vi "Image_Save_Handler_v_01.vi"(6 "Stop":bool, 8 "Sample+1":bool, 9 "Sample Name":string="Test Sample", 10 "Cam2":T2, 11 "Cam1":T2) -> (0 "Last Image?":bool, 2 "Image2":T1, 3 "Image1":T1)   [LabVIEW 2019]
doc: "Saves every 6th image in a sub folder in the current directory (specified from Sample Name). When a true is sent to Sample+1 a new subfolder is created with incremental numbering.\nExample of folders: \n../images/Sample_Name/Sample_Name1\n../images/Sample_Name/Sample_Name2"
uses:
  <extravilib>/ChannelInstances/Stream-t'IMAQ Image.ctl'/)Channel.ctl
  <vilib>/vision/Image Controls.llb/IMAQ Image.ctl
  <extravilib>/ChannelInstances/Stream-t'IMAQ Image.ctl'/Read With Abort.vi
  <extravilib>/ChannelInstances/Stream-t'IMAQ Image.ctl'/EndpointRead.vi
  <extravilib>/ChannelInstances/Stream-t'IMAQ Image.ctl'/)Channel.vi
  <resource>/ChannelSupport/_ChannelSupport/WaitIfNeeded.vi
  <extravilib>/ChannelInstances/Stream-t'IMAQ Image.ctl'.lvlib
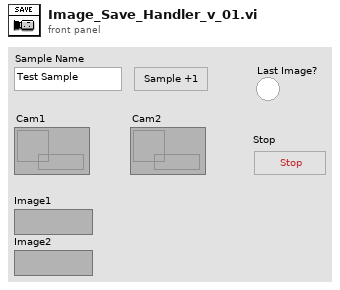
[diagram p1: front panel]
types:
  T1 = typedef "IMAQ Image.ctl" = refnum<image>
  T2 = typedef "Stream-t'IMAQ Image.ctl'.lvlib/)Channel.ctl" = refnum<queue>
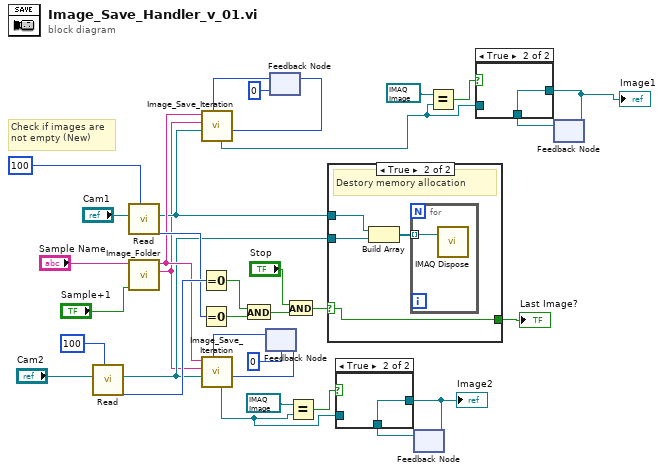
[diagram p0: block diagram]
diagram:
  # "Check if images are\nnot empty (New)"
  n1 = call <extravilib>:"Read.vi"("timeout in ms (-1)"=100, "channel"="Cam2") -> ("element"=w18:T1, "count"=w29:i32)  [unwired: 5 in, 3 out]
  n2 = call <extravilib>:"Read.vi"("timeout in ms (-1)"=100, "channel"="Cam1") -> ("element"=w19:T1, "count"=w21:i32)  [unwired: 5 in, 3 out]
  n3 = call "Image_Folder.vi"("New sample"="Sample+1", "Sample Name"="Sample Name") -> ("Subfolder Name"=w1:string, "Subfolder Path"=w20:string)  [unwired: 8 in]
  n4 = Equal To 0?(x=w29) -> (x = 0?=w24:bool)
  n5 = Equal To 0?(x=w21) -> (x = 0?=w23:bool)
  n6 = And(x=w24, y=w23) -> (x .and. y?=w22:bool)
  n7 = feedback #1(0 ("Iteration count out")) -> (w13:i32)
  n8 = call "Image_Save_Iteration.vi"("Iteration count in"=w13, "Image"=w18, "Subfolder Name"=w1, "Subfolder path"=w20) -> ("Iteration count out"=w14:i32, "Imageout"=w9:T1)  [unwired: 5 in, 1 out]
  n9 = feedback-in #1(w14) -> ()
  n10 = feedback #2(0 ("Iteration count out")) -> (w16:i32)
  n11 = call "Image_Save_Iteration.vi"("Iteration count in"=w16, "Image"=w19, "Subfolder Name"=w1, "Subfolder path"=w20) -> ("Iteration count out"=w17:i32, "Imageout"=w2:T1)  [unwired: 5 in, 1 out]
  n12 = feedback-in #2(w17) -> ()
  n13 = And(x="Stop", y=w22) -> (x .and. y?=w28:bool)
  n14 = Equal?(x=T1 refnum ("Image Out"), y=w9) -> (x = y?=w10:bool)
  n15 = case shown="True" w28 {
    selector: w28 -> [w35 w39]
    tunnel: [w35 w39] -> w26
    tunnel: w19 -> [_ w37]
    tunnel: w18 -> [_ w36]
    frame False {
    }
    frame True {
      # "Destory memory allocation"
      n16 = Build Array(w37, w36) -> (w38:T1[])
      n17 = for {
        tunnel: w38 -> [w40] mode=indexing
        n18 = call "IMAQ Dispose"("Image"=w40) -> ()  [unwired: 5 in, 1 out]
      }
    }
  }
  "Last Image?" <- w26
  n19 = feedback #3() -> (w8:T1)  [unwired: 1 in]
  n20 = case shown="True" w10 {
    tunnel: w9 -> [w41 _]
    tunnel: [w41 w42] -> w7
    tunnel: w8 -> [_ w42]
    frame False {
    }
    frame True {
    }
  }
  "Image2" <- w7
  n21 = feedback-in #3(w7) -> ()
  n22 = Equal?(x=T1 refnum ("Image Out"), y=w2) -> (x = y?=w5:bool)
  n23 = feedback #4() -> (w4:T1)  [unwired: 1 in]
  n24 = case shown="True" w5 {
    tunnel: w2 -> [w43 _]
    tunnel: [w43 w44] -> w3
    tunnel: w4 -> [_ w44]
    frame False {
    }
    frame True {
    }
  }
  "Image1" <- w3
  n25 = feedback-in #4(w3) -> ()
